vi "PatchCore_DS_Reader.vi"(4 "Read Options":T1, 6 "Good Unique Labels":string[](array[string]), 7 "PreProc_Options_in":T2={"DS_Name"="", "Input_Dims"={"C"=3, "H"=224, "W"=224}, "Center Crop Size"=0, "Interpolation Type"=1, "Multi-Stage_DownSample?"=FALSE, "Dataset_Stats"={"means"={"R"=0.5385, "G"=0.5348, "B"=0.551}, "stds"={"R"=0.3673, "G"=0.3673, "B"=0.3505}}} {"Dataset_Stats"."stds"."R" format="%#_3g"; "Dataset_Stats"."stds"."G" format="%#_3g"; "Dataset_Stats"."stds"."B" format="%#_3g"; "Dataset_Stats"."means"."R" format="%#_3g"; "Dataset_Stats"."means"."G" format="%#_3g"; "Dataset_Stats"."means"."B" format="%#_3g"; "Interpolation Type" items=["Zero Order", "Bi-Linear", "Quadratic", "Cubic Spline"]}, 8 "error in (no error)":errorcluster, 10 "GT Folder Path":path, 11 "Folder Path":path=path "D:/DNN/_AD/Ngene/AD_PCB3/00_Orig/test") -> (0 "error out":errorcluster, 1 "PreProc_Options_out":T2={"DS_Name"="00_Orig", "Input_Dims"={"C"=4, "H"=224, "W"=224}, "Center Crop Size"=0, "Interpolation Type"=1, "Multi-Stage_DownSample?"=FALSE, "Dataset_Stats"={"means"={"R"=0.5385, "G"=0.5348, "B"=0.551}, "stds"={"R"=0.3673, "G"=0.3673, "B"=0.3505}}} {"Dataset_Stats"."stds"."R" format="%#_3g"; "Dataset_Stats"."stds"."G" format="%#_3g"; "Dataset_Stats"."stds"."B" format="%#_3g"; "Dataset_Stats"."means"."R" format="%#_3g"; "Dataset_Stats"."means"."G" format="%#_3g"; "Dataset_Stats"."means"."B" format="%#_3g"; "Interpolation Type" items=["Zero Order", "Bi-Linear", "Quadratic", "Cubic Spline"]}, 3 "Dataset":T6={"Dataset_Size"=0, "Dims_In"={"C"=4, "H"=224, "W"=224}, "Labels"=[], "File Paths"=[], "Outputs Ref."=refnum, "Inputs Ref."=variant(refnum<data-value> refnum), "Dims_Out"={"C"=4, "H"=224, "W"=224}}, 5 "dT_DS_Reader":dbl=0.03407189999416005)   [LabVIEW 2024]
uses:
  <vilib>/Ngene/Deep Learning Toolkit/Toolkit/NN_Data/API/DataSet/DataSet_Types/NN_DataSet(In3D_Out3D).ctl
  <vilib>/Ngene/Deep Learning Toolkit/Toolkit/NN_Data/API/NN_Dims(C,H,W).ctl
  <vilib>/Ngene/Deep Learning Toolkit/Toolkit/NN_Data/Controls/DataRef_Types/4D/NN_Data_ref(4D_SGL).ctl
  <vilib>/Ngene/DeepLTK Anomaly Detection Addon/DeepLTK_Anomaly_Detection_Addon/API/Controls/NNPC_PreProcessing_Options.ctl
  <vilib>/Ngene/DeepLTK Anomaly Detection Addon/DeepLTK_Anomaly_Detection_Addon/API/Controls/NNPC_DS_Stats.ctl
  <vilib>/Ngene/DeepLTK Anomaly Detection Addon/DeepLTK_Anomaly_Detection_Addon/API/Controls/Image_Stats_RGB.ctl
  Controls/Read_Options.ctl
  <vilib>/Ngene/Deep Learning Toolkit/Toolkit/Deep_Learning_Toolkit_by_Ngene.lvlib
  <vilib>/vision/NI_Vision_Development_Module.lvlib
  <vilib>/Ngene/DeepLTK Anomaly Detection Addon/DeepLTK_Anomaly_Detection_Addon/DeepLTK_Anomaly_Detection_Addon.lvlib
panel:
  out "Numeric":i32
  out "Progress":i32
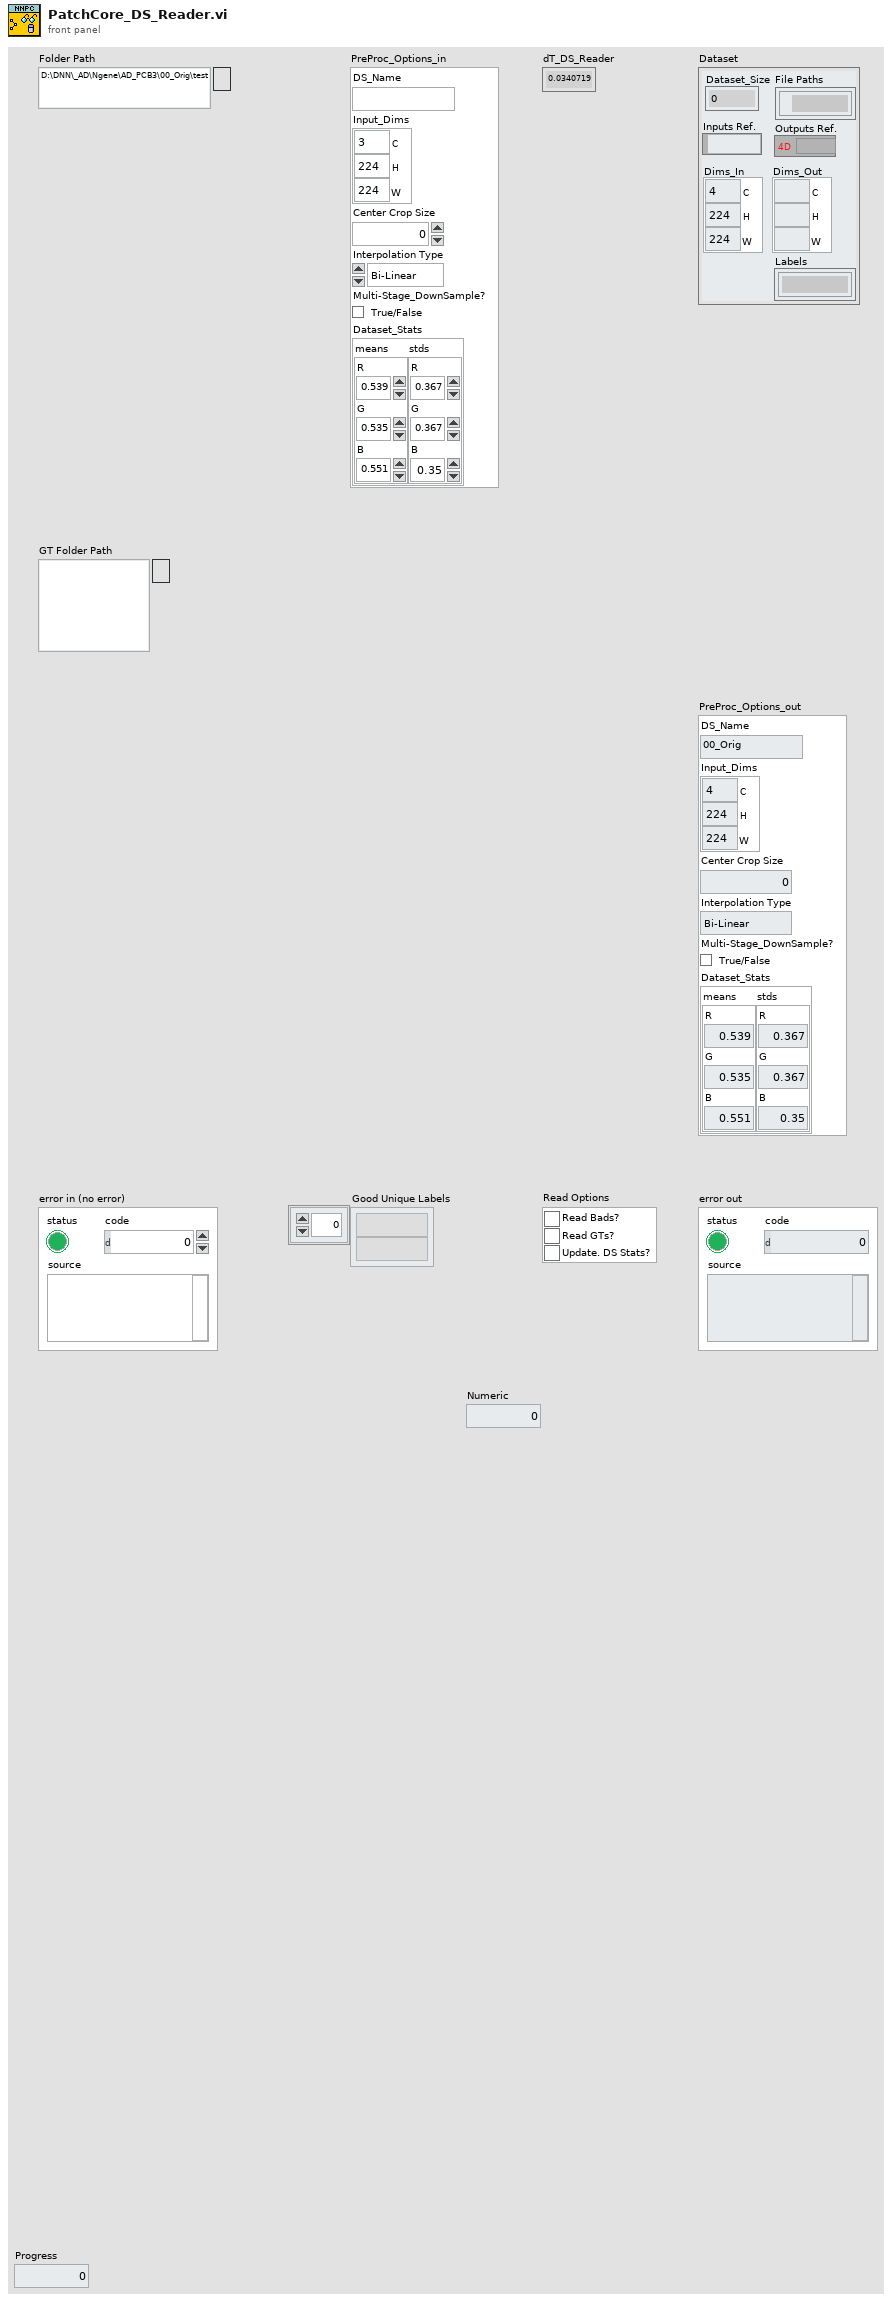
[diagram p1: front panel]
types:
  T1 = typedef "Read_Options.ctl" = cluster{"Read Bads?":bool, "Read GTs?":bool, "Update. DS Stats?":bool}
  T2 = typedef "DeepLTK_Anomaly_Detection_Addon.lvlib/NNPC_PreProcessing_Options.ctl" = cluster{"DS_Name":string, "Input_Dims":T3, "Center Crop Size":i32, "Interpolation Type":u32, "Multi-Stage_DownSample?":bool, "Dataset_Stats":T4}
  T3 = typedef "Deep_Learning_Toolkit_by_Ngene.lvlib/NN_Dims(C,H,W).ctl" = cluster{"C":i32, "H":i32, "W":i32}
  T4 = typedef "DeepLTK_Anomaly_Detection_Addon.lvlib/NNPC_DS_Stats.ctl" = cluster{"means":T5, "stds":T5}
  T5 = typedef "DeepLTK_Anomaly_Detection_Addon.lvlib/Image_Stats_RGB.ctl" = cluster{"R":sgl, "G":sgl, "B":sgl}
  T6 = typedef "Deep_Learning_Toolkit_by_Ngene.lvlib/NN_DataSet(In3D_Out3D).ctl" = cluster{"Dataset_Size":i32, "Dims_In":T3, "Labels":string[], "File Paths":path[], "Outputs Ref.":T7, "Inputs Ref.":variant, "Dims_Out":T3}
  T7 = typedef "Deep_Learning_Toolkit_by_Ngene.lvlib/NN_Data_ref(4D_SGL).ctl" = refnum<data-value>
  T8 = typedef "Image Type" = u32
  T9 = typedef "IMAQ Image.ctl" = refnum<image>
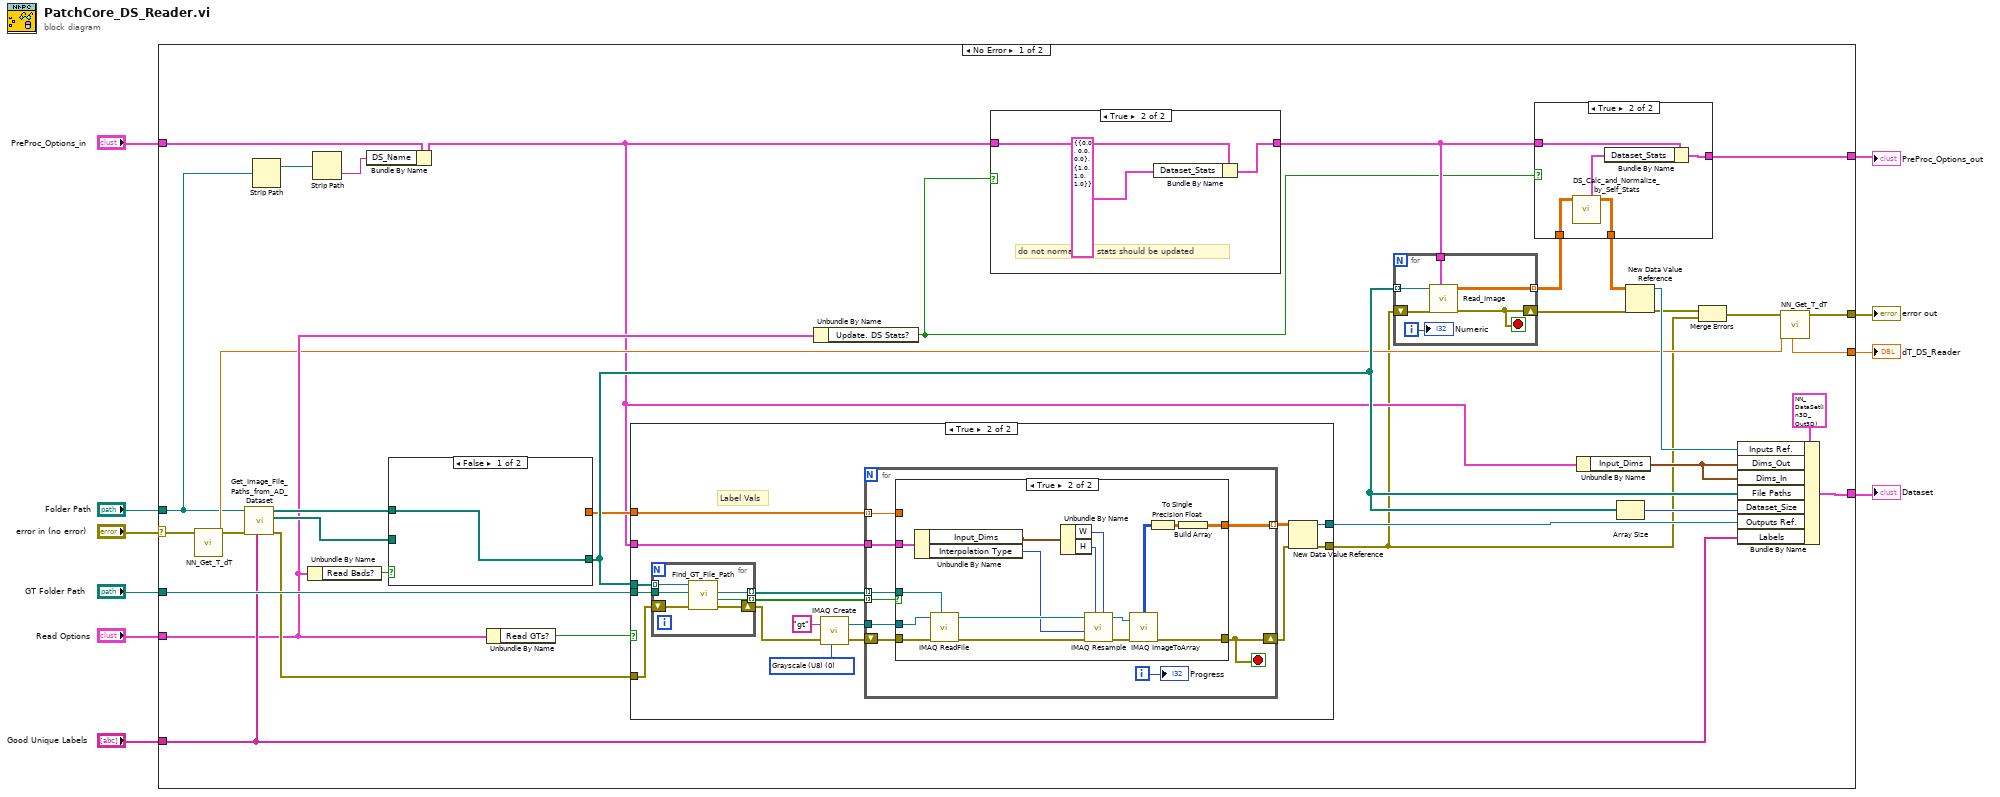
[diagram p0: block diagram]
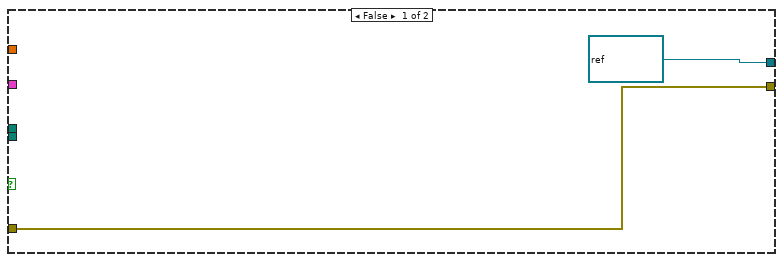
[diagram p2: hidden frame]
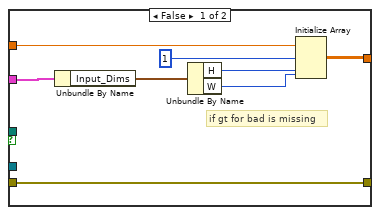
[diagram p3: hidden frame]
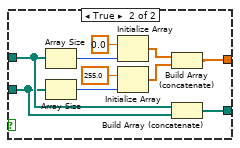
[diagram p4: hidden frame]
diagram:
  n1 = case shown="No Error" "error in (no error)" {
    selector: "error in (no error)" -> [w45 w131]
    tunnel: [w44 _] -> w9
    tunnel: "GT Folder Path" -> [w41 _]
    tunnel: "Good Unique Labels" -> [w39 _]
    tunnel: "Read Options" -> [w30 _]
    tunnel: [w27 w131] -> w5
    tunnel: [w25 _] -> w4
    tunnel: "Folder Path" -> [w24 _]
    tunnel: "PreProc_Options_in" -> [w21 _]
    tunnel: [w12 _] -> w1
    frame No Error {
      n2 = call <vilib>:"NN_Get_T_dT.vi"("error in (no error)"=w45) -> ("T_out"=w26:dbl, "error out"=w28:errorcluster)  [unwired: 6 in, 1 out]
      n3 = call "Get_Image_File_Paths_from_AD_Dataset.vi"("Good Folder Names"=w39, "error in"=w28, "Dataset Folder"=w24) -> ("error out"=w32:errorcluster, "Bad Dataset Files"=w38:path[], "Good Dataset Files"=w37:path[])  [unwired: 6 in]
      n4 = Strip Path(path=w24) -> (stripped path=w23:path)  [unwired: 1 out]
      n5 = Unbundle By Name(w30) -> ("Read Bads?"=w34:bool)
      n6 = Strip Path(path=w23) -> (name=w19:string)  [unwired: 1 out]
      n7 = Bundle By Name(cluster=w21, "DS_Name"=w19) -> (w20:T2)
      n8 = case shown="False" w34 {
        tunnel: w37 -> [w103 w112]
        tunnel: [w103 w113] -> w36
        tunnel: w38 -> [_ w107]
        tunnel: [_ w104] -> w35
        frame False {
        }
        frame True {
          n9 = Array Size(array=w112) -> (size(s)=w111:i32)
          n10 = Array Size(array=w107) -> (size(s)=w108:i32)
          n11 = Initialize Array(sgl 0.0 ("element"), w111) -> (w106:sgl[])
          n12 = Initialize Array(sgl 255.0 ("element"), w108) -> (w105:sgl[])
          n13 = Build Array (concatenate)(w106, w105) -> (w104:sgl[])
          n14 = Build Array (concatenate)(w112, w107) -> (w113:path[])
        }
      }
      n15 = Unbundle By Name(w30) -> ("Read GTs?"=w33:bool)
      n16 = case shown="True" w33 {
        tunnel: w32 -> [w47 w50]
        tunnel: [refnum<data-value> refnum ("data value reference") w57] -> w42
        tunnel: w41 -> [_ w55]
        tunnel: [w47 w54] -> w11
        tunnel: w36 -> [_ w53]
        tunnel: w35 -> [_ w51]
        tunnel: w20 -> [_ w48]
        frame False {
        }
        frame True {
          w59 = T8 0 items=["Grayscale (U8)", "Grayscale (I16)", "Grayscale (SGL)", "Complex (CSG)", "RGB (U32)", "HSL (U32)", "RGB (U64)", "Grayscale (U16)"] ("Image Type")
          # "Label Vals"
          n17 = for {
            tunnel: w55 -> [w69]
            tunnel: w53 -> [w66] mode=indexing
            tunnel: [w67] -> w56 mode=indexing
            tunnel: [w68] -> w52 mode=indexing
            shift-right: [w64] -> w49
            shift-left: w50 -> [w65]
            n18 = call "Find_GT_File_Path.vi"("error in"=w65, "GT Mask Folder Path"=w69, "Image File Path"=w66) -> ("error out"=w64:errorcluster, "Found?"=w68:bool, "GT File Path"=w67:path)  [unwired: 5 in, 1 out]
          }
          n19 = call "IMAQ Create"("Image Name"="gt", "Image Type"=w59, "error in (no error)"=w49) -> ("New Image"=w63:T9, "error out"=w61:errorcluster)  [unwired: 2 in]
          n20 = for {
            tunnel: w63 -> [w78]
            tunnel: w56 -> [w76] mode=indexing
            tunnel: [w75] -> w58 mode=indexing
            shift-right: [w73] -> w60
            shift-left: w61 -> [w77]
            tunnel: w52 -> [w72] mode=indexing
            tunnel: w51 -> [w71] mode=indexing
            tunnel: w48 -> [w70]
            i -> [w74]
            stop <- w73 stop-if-true
            n21 = case shown="True" w72 {
              tunnel: w78 -> [_ w102]
              tunnel: w77 -> [w84 w101]
              tunnel: w76 -> [_ w100]
              tunnel: [w85 w99] -> w75
              tunnel: [w84 w95] -> w73
              tunnel: w71 -> [w81 _]
              tunnel: w70 -> [w79 w87]
              frame False {
                # "if gt for bad is missing"
                n22 = Unbundle By Name(w79) -> ("Input_Dims"=w80:T3)
                n23 = Unbundle By Name(w80) -> ("H"=w82:i32, "W"=w83:i32)
                n24 = Initialize Array(w81, 1 ("dimension size"), w82, w83) -> (w85:sgl[][][])
              }
              frame True {
                n25 = Unbundle By Name(w87) -> ("Input_Dims"=w89:T3, "Interpolation Type"=w88:u32)
                n26 = call "IMAQ ReadFile"("File Path"=w100, "error in (no error)"=w101, "Image"=w102) -> ("error out"=w93:errorcluster, "Image Out"=w92:T9)  [unwired: 4 in, 3 out]
                n27 = Unbundle By Name(w89) -> ("W"=w91:i32, "H"=w90:i32)
                n28 = call "IMAQ Resample"("X Resolution"=w91, "Y Resolution"=w90, "error in (no error)"=w93, "Interpolation Type"=w88, "Image Src"=w92) -> ("error out"=w97:errorcluster, "Image Dst Out"=w98:T9)  [unwired: 5 in]
                n29 = call "IMAQ ImageToArray"("error in (no error)"=w97, "Image"=w98) -> ("error out"=w95:errorcluster, "Image Pixels (U8)"=w94:u8[][])  [unwired: 2 in, 3 out]
                n30 = To Single Precision Float(number=w94) -> (single precision float=w96:sgl[][])
                n31 = Build Array(w96) -> (w99:sgl[][][])
              }
            }
            "Progress" <- w74
          }
          n32 = New Data Value Reference(data value=w58, error in=w60) -> (data value reference=w57:refnum<data-value>, error out=w54:errorcluster)
        }
      }
      n33 = Unbundle By Name(w30) -> ("Update. DS Stats?"=w13:bool)
      n34 = case shown="True" w13 {
        tunnel: w20 -> [w114 w117]
        tunnel: [w114 w115] -> w15
        frame False {
        }
        frame True {
          # "do not normalize if stats should be updated"
          n35 = Bundle By Name(cluster=w117, "Dataset_Stats"=T4 {"means"={"R"=0.0, "G"=0.0, "B"=0.0}, "stds"={"R"=1.0, "G"=1.0, "B"=1.0}}) -> (w115:T2)
        }
      }
      n36 = for {
        tunnel: [w119] -> w16 mode=indexing
        tunnel: w15 -> [w120]
        tunnel: w36 -> [w121] mode=indexing
        shift-right: [w122] -> w17
        shift-left: w11 -> [w123]
        i -> [w118]
        stop <- w122 stop-if-true
        n37 = call "Read_Image.vi"("PreProcessing_Options"=w120, "error in"=w123, "Img Path"=w121) -> ("error out"=w122:errorcluster, "Image Out"=w119:sgl[][][])  [unwired: 5 in, 2 out]
        "Numeric" <- w118
      }
      n38 = case shown="True" w13 {
        tunnel: w16 -> [w125 w128]
        tunnel: [w125 w126] -> w14
        tunnel: w15 -> [w124 w130]
        tunnel: [w124 w129] -> w12
        frame False {
        }
        frame True {
          n39 = call "DS_Calc_and_Normalize_by_Self_Stats.vi"("DS in"=w128) -> ("DS out"=w126:sgl[][][][], "Dataset_Stats"=w127:T4)  [unwired: 9 in]
          n40 = Bundle By Name(cluster=w130, "Dataset_Stats"=w127) -> (w129:T2)
        }
      }
      n41 = Unbundle By Name(w20) -> ("Input_Dims"=w22:T3)
      n42 = Array Size(array=w36) -> (size(s)=w29:i32)
      n43 = New Data Value Reference(data value=w14, error in=w17) -> (data value reference=w31:refnum<data-value>, error out=w18:errorcluster)
      n44 = Merge Errors(w18, w11) -> (w40:errorcluster)
      n45 = Bundle By Name(cluster=T6 {"Dataset_Size"=0, "Dims_In"={"C"=0, "H"=0, "W"=0}, "Labels"=[], "File Paths"=[], "Outputs Ref."=refnum, "Inputs Ref."=variant, "Dims_Out"={"C"=0, "H"=0, "W"=0}} ("Dataset(In3D_Out3D)"), "Inputs Ref."=w31, "Dims_Out"=w22, "Dims_In"=w22, "File Paths"=w36, "Dataset_Size"=w29, "Outputs Ref."=w42, "Labels"=w39) -> (w44:T6)
      n46 = call <vilib>:"NN_Get_T_dT.vi"("T_in"=w26, "error in (no error)"=w40) -> ("error out"=w27:errorcluster, "dT"=w25:dbl)  [unwired: 5 in, 1 out]
    }
    frame Error {
    }
  }
  "error out" <- w5
  "Dataset" <- w9
  "dT_DS_Reader" <- w4
  "PreProc_Options_out" <- w1
